vi "SetChoose2Position.vi"(0 "Choose2":refnum<vi>, 1 "Mode":refnum<vi>, 2 "Pane Refnum":refnum<vi>) -> ()   [LabVIEW 2014]
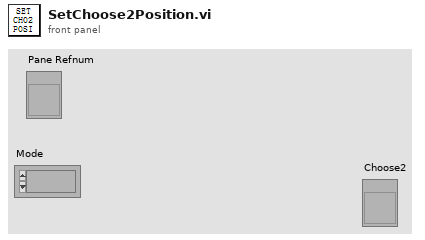
[diagram p1: front panel]
types:
  T1 = typedef "LVRectTypeDef.ctl" = cluster{"Left":i16, "Top":i16, "Right":i16, "Bottom":i16}
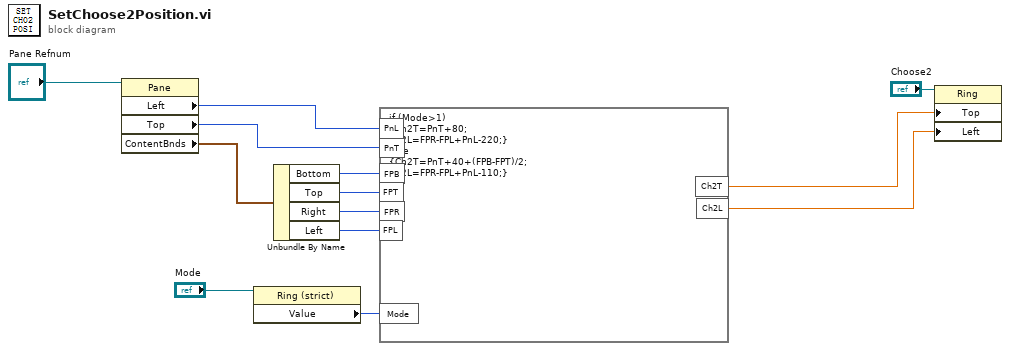
[diagram p0: block diagram]
diagram:
  n1 = property class="Pane"(reference="Pane Refnum") -> ("Left"=w2:i32, "Top"=w1:i32, "ContentBnds"=w3:T1)  [unwired: 1 in, 2 out]
  n2 = property class="Ring (strict)"(reference="Mode") -> ("Value"=w4:u16)  [unwired: 1 in, 2 out]
  n3 = Unbundle By Name(w3) -> ("Bottom"=w11:i16, "Top"=w10:i16, "Right"=w9:i16, "Left"=w8:i16)
  n4 = formula code="if (Mode>1)\n{Ch2T=PnT+80;\nCh2L=FPR-FPL+PnL-220;}\nelse\n{Ch2T=PnT+40+(FPB-FPT)/2;\nCh2L=FPR-FPL+PnL-110;}"("FPB"=w11, "FPT"=w10, "FPR"=w9, "FPL"=w8, "PnT"=w1, "PnL"=w2, "Mode"=w4) -> ("Ch2T"=w7:dbl, "Ch2L"=w6:dbl)
  n5 = property class="Ring"(reference="Choose2", "Top"=w7, "Left"=w6) -> ()  [unwired: 1 in, 2 out]
